vi "test_TCP_constants_letters_start.vi"() -> (1 "output_byte_uppercase":u8=60, 2 "output_byte_lowercase":u8=60)   [LabVIEW 2014]
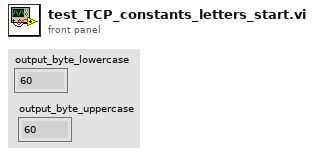
[diagram p1: front panel]
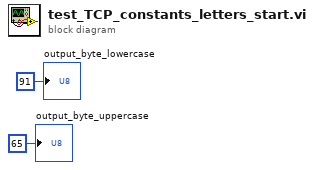
[diagram p0: block diagram]
diagram:
  "output_byte_lowercase" <- u8 91
  "output_byte_uppercase" <- u8 65
